vi "Destroy ProgressBar.vi"(8 "error in (no error)":errorcluster, 11 "ProgressBar in":refnum<class "ProgressBar.lvclass">) -> (0 "error out":errorcluster, 3 "ProgressBar out":refnum<class "ProgressBar.lvclass">)   [LabVIEW 2019, in "ProgressBar.lvclass"]
uses:
  ProgressBar.lvclass
  C:/Program Files (x86)/National Instruments/LabVIEW 2019/vi.lib/JKI/JKI SMO/SMO/SMO.lvclass
  <vilib>/JKI/JKI SMO/SMO/SMO.lvclass
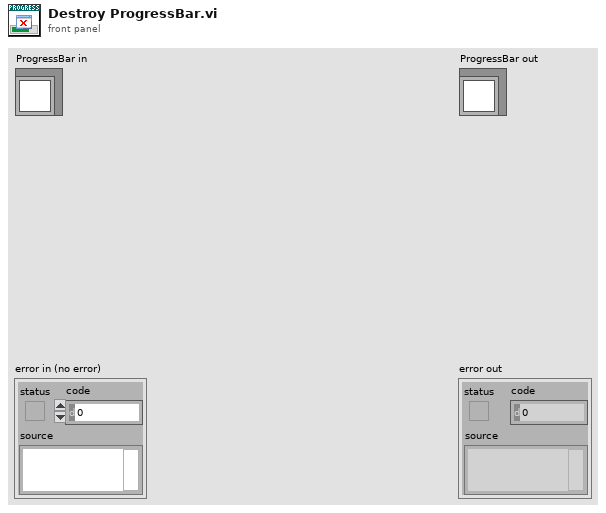
[diagram p1: front panel]
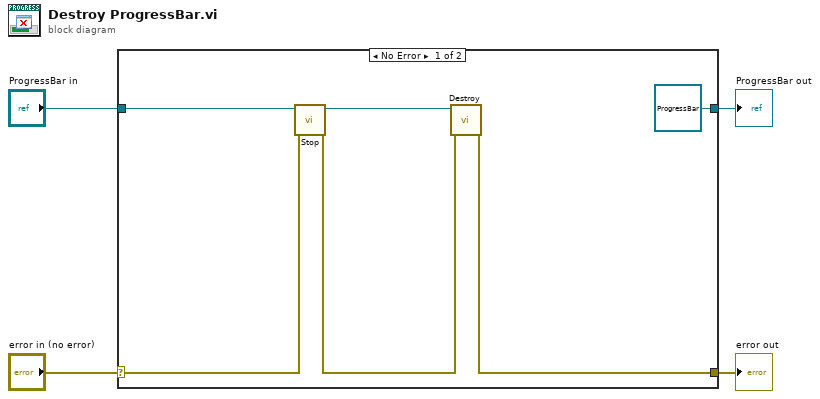
[diagram p0: block diagram]
diagram:
  n1 = case shown="No Error" "error in (no error)" {
    selector: "error in (no error)" -> [w7 w12]
    tunnel: [w9 w12] -> w3
    tunnel: [refnum<class "ProgressBar.lvclass"> refnum ("ProgressBar in") w11] -> w1
    tunnel: "ProgressBar in" -> [w6 w11]
    frame No Error {
      n2 = call <vilib>:"Stop.vi"("error in (no error)"=w7, "SMO"=w6) -> ("error out"=w8:errorcluster, "SMO out"=w5:refnum<class "ProgressBar.lvclass">)  [unwired: 8 in]
      n3 = call <vilib>:"Destroy.vi"("error in (no error)"=w8, "SMO"=w5) -> ("error out"=w9:errorcluster)  [unwired: 9 in]
    }
    frame Error {
    }
  }
  "error out" <- w3
  "ProgressBar out" <- w1
